vi "Launch Root State Actor.vi"(4 "Debug Alias":string, 6 "Open Actor Core front panel? (F)":bool, 8 "error in (no error)":errorcluster, 10 "State Actor":refnum<class "State Actor.lvclass">) -> (0 "error out":errorcluster, 1 "State Transition User Event":refnum<user-event>, 2 "Actor's Enqueuer":refnum<class "Message Enqueuer.lvclass">)   [LabVIEW 2024, in "State Actor.lvlib" / "State Actor.lvclass"]
uses:
  State Actor.lvclass
  C:/Program Files (x86)/National Instruments/LabVIEW 2024/vi.lib/ActorFramework/Actor/Actor.lvclass
  <vilib>/ActorFramework/Message Enqueuer/Message Enqueuer.lvclass
  State Actor Messages/Get State Transition User Event Msg/Get State Transition User Event Msg.lvclass/Get State Transition User Event Msg.ctl
  <vilib>/ActorFramework/Message Enqueuer/Message Enqueuer.lvclass/Message Enqueuer.ctl
  <vilib>/ActorFramework/Message Enqueuer/Enqueue.vi
  State Actor Messages/Get State Transition User Event Msg/Get State Transition User Event Msg.lvclass
  C:/Program Files (x86)/National Instruments/LabVIEW 2024/vi.lib/ActorFramework/Message/Message.lvclass
  <vilib>/ActorFramework/Message Priority Queue/Priority Enqueue.vi
  State Actor.lvclass/State Actor.ctl
  <vilib>/ActorFramework/Actor/Actor.lvclass
  State Transition Event.ctl
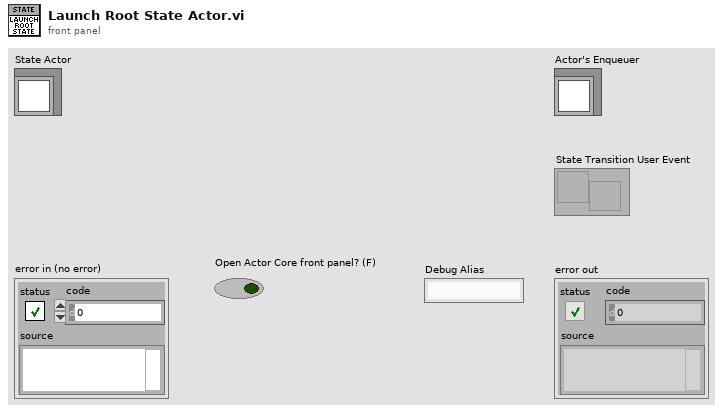
[diagram p1: front panel]
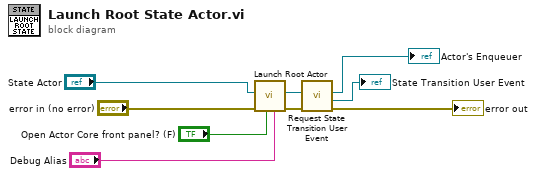
[diagram p0: block diagram]
diagram:
  n1 = call <vilib>:"Launch Root Actor.vi"("Debug Alias"="Debug Alias", "Open Actor Core front panel? (F)"="Open Actor Core front panel? (F)", "error in (no error)"="error in (no error)", "Actor"="State Actor") -> ("error out"=w2:errorcluster, "Actor's Enqueuer"=w3:refnum<class "Message Enqueuer.lvclass">)  [unwired: 6 in]
  n2 = call "Request State Transition User Event.vi"("error in (no error)"=w2, "Message Enqueuer"=w3) -> ("error out"=→"error out":errorcluster, "State Transition User Event"=→"State Transition User Event":refnum<user-event>, "Message Enqueuer out"=→"Actor's Enqueuer":refnum<class "Message Enqueuer.lvclass">)  [unwired: 7 in]
